vi "testing_file.vi"() -> ()   [LabVIEW 2017]
uses:
  UI Error Handlers/support/Logging/Logging.lvlib
panel:
  in  "Boolean 2":bool
  in  "Boolean":bool
  out "AVI Path":path
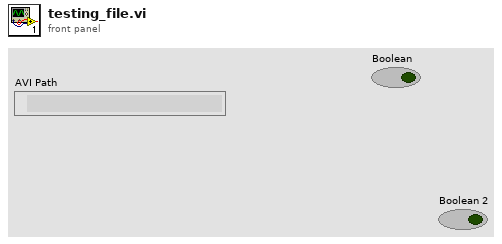
[diagram p1: front panel]
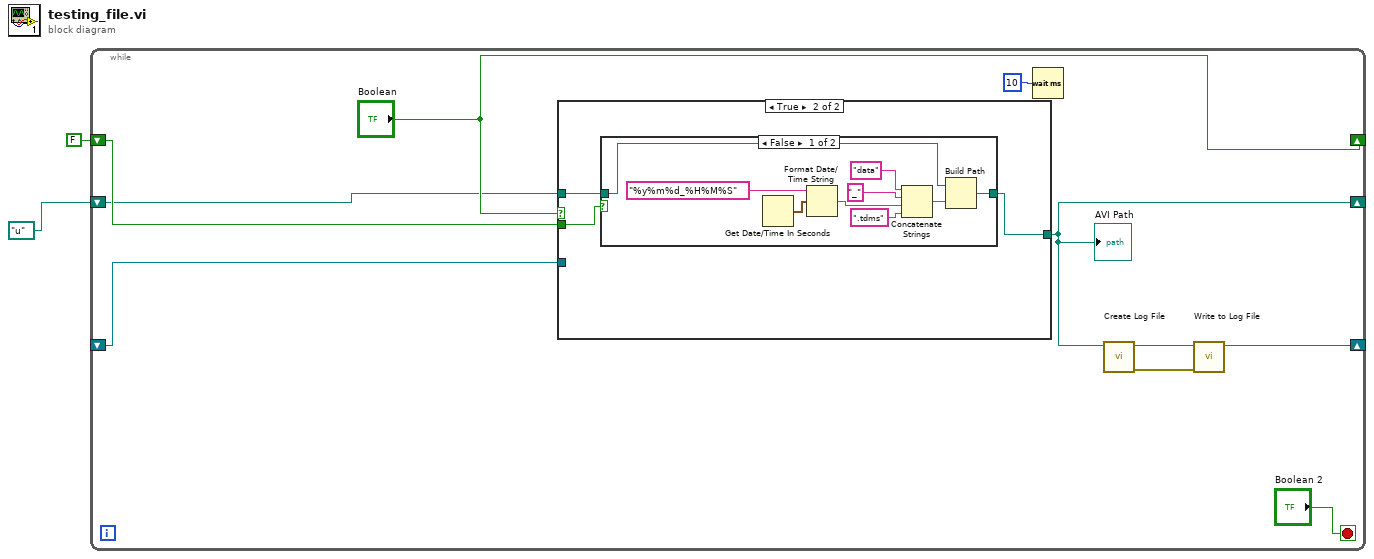
[diagram p0: block diagram]
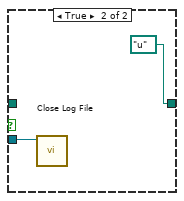
[diagram p3: hidden frame]
diagram:
  n1 = while {
    shift-right: ["Boolean"] -> _
    shift-left: FALSE ("Boolean") -> [w7]
    shift-right: [w6] -> _
    shift-left: path "u:/" ("AVI Path") -> [w5]
    shift-right: [w4] -> _
    shift-left: _ -> [w3]
    stop <- "Boolean 2" stop-if-true
    n2 = case shown="True" "Boolean" {
      tunnel: [w14 w22] -> w6
      tunnel: w7 -> [w15 w21]
      tunnel: w5 -> [w13 w20]
      tunnel: w3 -> [w16 _]
      frame False {
        n3 = case shown="False" w15 {
          tunnel: w16 -> [_ w19]
          tunnel: w13 -> [w17 _]
          tunnel: [w17 path "u:/" ("AVI Path")] -> w14
          frame False {
          }
          frame True {
            n4 = call "Close Log File.vi"("tdms file"=w19) -> ()  [unwired: 10 in, 1 out]
          }
        }
      }
      frame True {
        n5 = case shown="False" w21 {
          tunnel: [w24 w32] -> w22
          tunnel: w20 -> [w23 w32]
          frame False {
            n6 = Get Date/Time In Seconds() -> (seconds since 1Jan1904=w27:timestamp)
            n7 = Format Date/Time String(time format string (%c)="%y%m%d_%H%M%S", seconds (now)=w27) -> (date/time string=w30:string)  [unwired: 1 out]
            n8 = Concatenate Strings("data" ("string"), "_" ("string"), w30, ".tdms" ("string")) -> (w25:string)
            n9 = Build Path(base path=w23, name or relative path=w25) -> (appended path=w24:path)
          }
          frame True {
          }
        }
      }
    }
    "AVI Path" <- w6
    n10 = Wait (ms)(milliseconds to wait=u32 10) -> ()  [unwired: 1 out]
    n11 = call "Create Log File.vi"("Acceleration Exceeded Log Folder"=w6) -> ("error out"=w12:errorcluster, "Log File out"=w11:refnum<k34>)  [unwired: 9 in]
    n12 = call "Write to Log File.vi"("error in (no error)"=w12, "Log File in"=w11) -> ("Log File out"=w4:refnum<k34>)  [unwired: 8 in, 1 out]
  }
